vi "Flush To Disk.vi"(8 "error in (no error)":errorcluster) -> (0 "error out":errorcluster)   [LabVIEW 2020, in "Logger.lvlib"]
uses:
  Logger.lvlib
  LoggerGlobal.vi
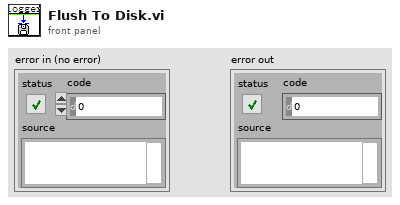
[diagram p1: front panel]
types:
  T1 = enum16{"open", "replace", "create", "open or create", "replace or create", "replace or create with confirmation"}
  T2 = typedef "Event.ctl" = cluster{"Time":string, "Event":string, "Information":string}
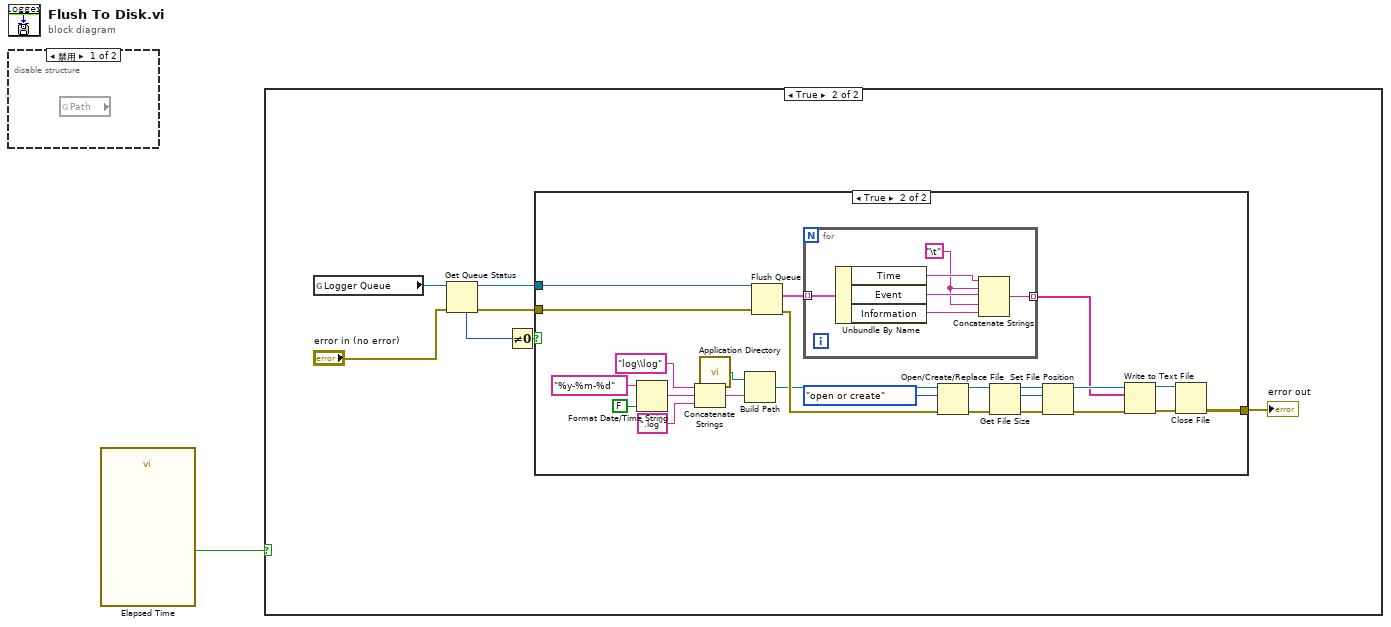
[diagram p0: block diagram]
diagram:
  n1 = disable-structure shown="禁用" {
    frame Disabled {
      n2 = global read "LoggerGlobal.vi" "Path"() -> ()  [unwired: 1 out]
    }
    frame Enabled {
    }
  }
  n3 = call "Elapsed Time"() -> ("Time has Elapsed"=w1:bool)  [unwired: 12 in, 7 out]
  n4 = case shown="True" w1 {
    frame False {
    }
    frame True {
      n5 = global read "LoggerGlobal.vi" "Logger Queue"() -> (w8:refnum<queue>)
      n6 = Get Queue Status(queue=w8, error in (no error)="error in (no error)") -> (queue out=w5:refnum<queue>, error out=w4:errorcluster, # elements in queue=w6:i32)  [unwired: 1 in, 5 out]
      n7 = Not Equal To 0?(x=w6) -> (x != 0?=w3:bool)
      n8 = case shown="True" w3 {
        tunnel: w5 -> [_ w33]
        tunnel: w4 -> [w9 w32]
        tunnel: [w9 w18] -> w2
        frame False {
        }
        frame True {
          n9 = Format Date/Time String(time format string (%c)="%y-%m-%d" ("时间格式字符串(%c)"), UTC format=FALSE ("UTC格式")) -> (date/time string=w16:string)  [unwired: 1 in]
          n10 = Concatenate Strings("log\\log" ("名称或相对路径"), w16, ".log" ("字符串")) -> (w17:string)
          n11 = call <vilib>:"Application Directory.vi"() -> ("Application Directory"=w15:path)
          n12 = Build Path(base path=w15, name or relative path=w17) -> (appended path=w10:path)
          n13 = Flush Queue(queue=w33, error in (no error)=w32) -> (remaining elements=w24:T2[], error out=w23:errorcluster)  [unwired: 1 out]
          n14 = for {
            tunnel: w24 -> [w39] mode=indexing
            tunnel: [w34] -> w22 mode=indexing
            w36 = "\t"
            n15 = Unbundle By Name(w39) -> ("Time"=w38:string, "Event"=w37:string, "Information"=w35:string)
            n16 = Concatenate Strings(w38, w36, w37, w36, w35) -> (w34:string)
          }
          n17 = Open/Create/Replace File(file path (use dialog)=w10, error in=w23, operation (0:open)=T1."open or create") -> (refnum out=w29:refnum<file>, error out=w30:errorcluster)  [unwired: 3 in, 1 out]
          n18 = Get File Size(file=w29, error in=w30) -> (refnum out=w28:refnum<file>, size (in bytes)=w19:i64, 0:w27:errorcluster)
          n19 = Set File Position(offset (in bytes) (0)=w19, refnum=w28, error in=w27) -> (refnum out=w25:refnum<file>, error out=w26:errorcluster)  [unwired: 1 in]
          n20 = Write to Text File(file (use dialog)=w25, text=w22, error in=w26) -> (refnum out=w20:refnum<file>, error out=w21:errorcluster)  [unwired: 1 in, 1 out]
          n21 = Close File(refnum=w20, error in=w21) -> (error out=w18:errorcluster)  [unwired: 1 out]
        }
      }
      "error out" <- w2
    }
  }
